vi "resizable_alert_Main.vi"() -> ()   [LabVIEW 2016]
doc: "This template is for the Queued Message Handler design pattern.\n\nThe Event Handling Loop generates messages based on user interface actions.\n\nThe Message Handling Loop processes messages generated by the Event Handling Loop, or by other messages. The messages are string values, so new messages can be added easily to the Message Cases case structure in the Message Handling Loop. Each message cluster can also provide an optional value for Message Data, which is a variant that can be converted to whatever message-specific data is required."
uses:
  controls/resizable_alert_UI Data.ctl
  support/Message Queue/resizable_alert_Message Queue.lvlib
  <vilib>/Utility/error.llb/Error Cluster From Error Code.vi
  support/User Event - Stop/resizable_alert_User Event - Stop.lvlib
  support/Message Queue/Enqueue Message (Single).vi
  <vilib>/ErrorRing/Error Ring.xnode
panel:
  in  "header":string="Header Text"
  in  "explanatory text":string="A brief explanation of what happened and what you can do next."
  in  "close":bool
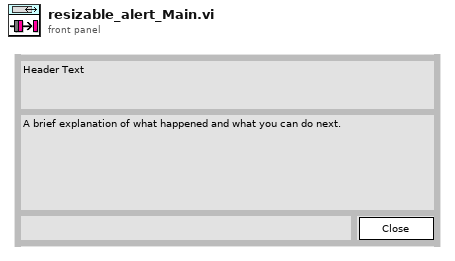
[diagram p1: front panel]
types:
  T1 = typedef "resizable_alert_UI Data.ctl" = cluster{"Exit Button Ref":refnum<vi>}
  T2 = typedef "resizable_alert_Message Queue.lvlib/All Message Queues.ctl" = cluster{"UI":refnum<queue>}
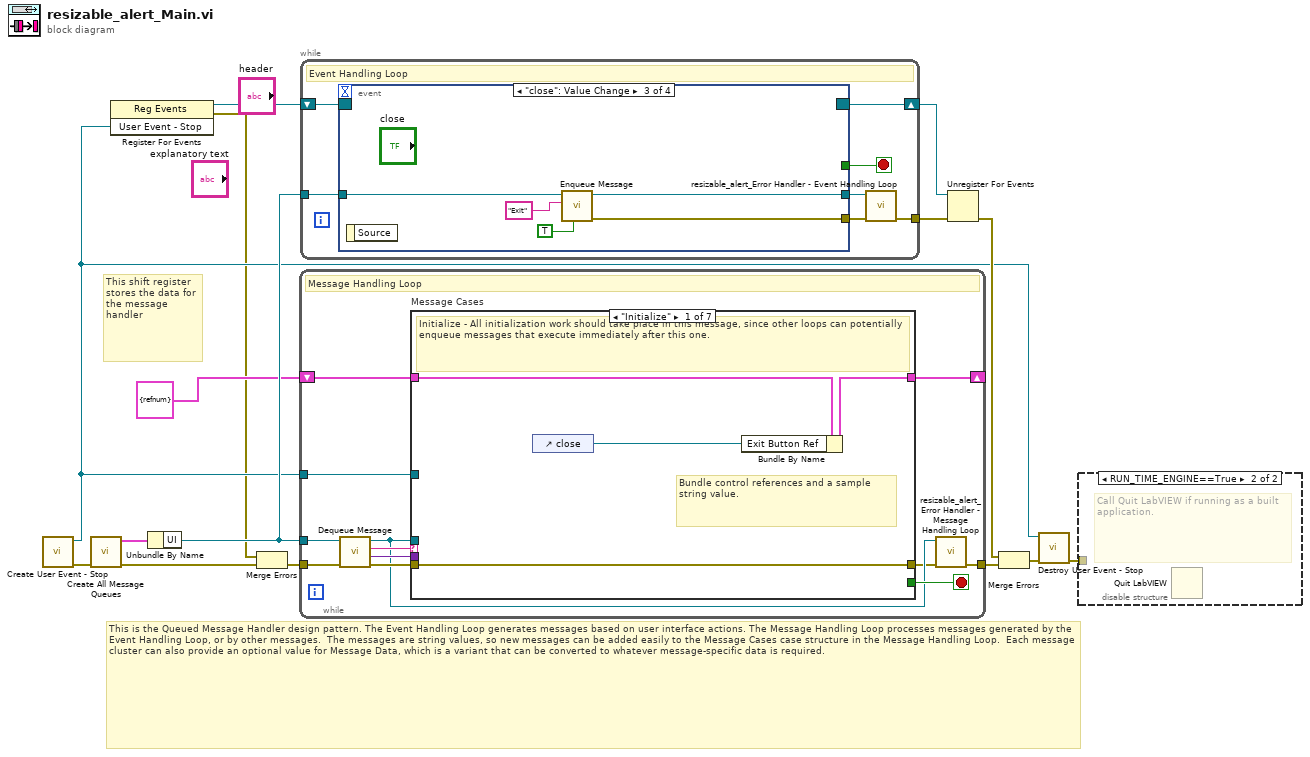
[diagram p0: block diagram]
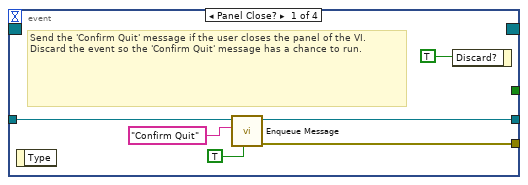
[diagram p3: hidden frame]
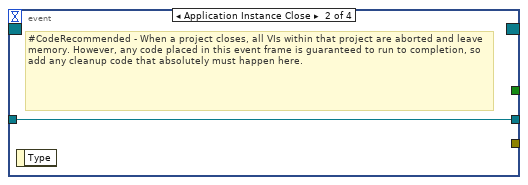
[diagram p4: hidden frame]
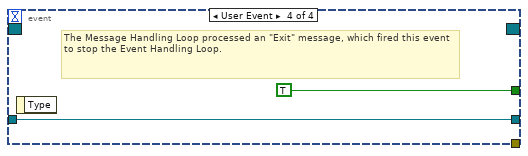
[diagram p5: hidden frame]
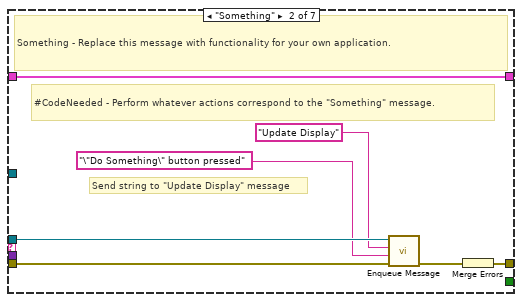
[diagram p6: hidden frame]
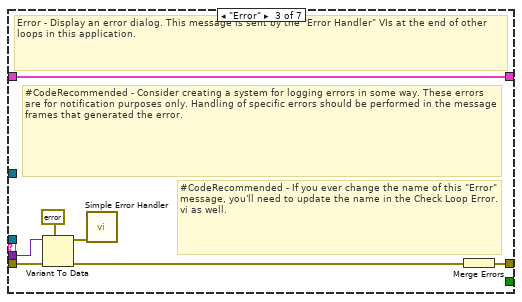
[diagram p7: hidden frame]
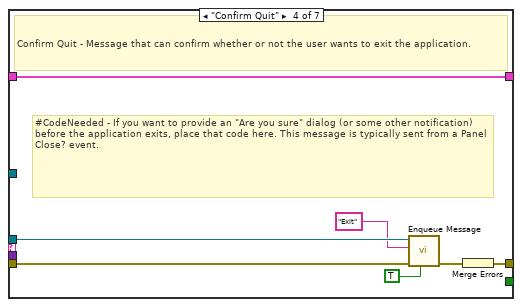
[diagram p8: hidden frame]
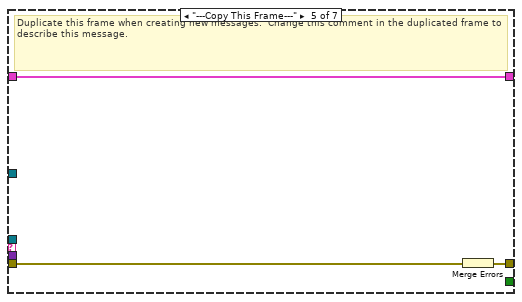
[diagram p9: hidden frame]
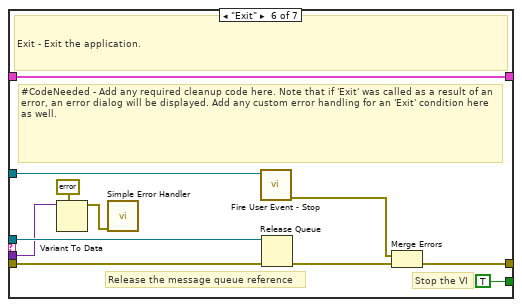
[diagram p10: hidden frame]
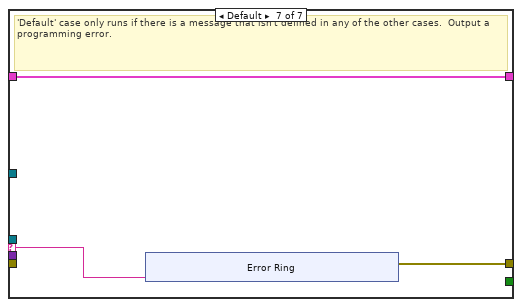
[diagram p11: hidden frame]
diagram:
  # "This is the Queued Message Handler design pattern. The Event Handling Loop generates messages based on user interface actions. The Message Handling Loop processes messages generated by the Event Handling Loop, or by other messages.  The messages are string values, so new messages can be added easily to the Message Cases case structure in the Message Handling Loop.  Each message cluster can also provide an optional value for Message Data, which is a variant that can be converted to whatever message-specific data is required."
  # "This shift register stores the data for the message handler"
  n1 = call "Create User Event - Stop.vi"() -> ("error out"=w11:errorcluster, "User Event - Stop"=w3:refnum<user-event>)  [unwired: 10 in]
  n2 = call "Create All Message Queues.vi"("error in (no error)"=w11) -> ("error out"=w15:errorcluster, "Message Queues out"=w14:T2)  [unwired: 9 in]
  n3 = register-events(w3) -> (reference out=w4:refnum<event-registration>, error out=w1:errorcluster)  [unwired: 2 in]
  n4 = Unbundle By Name(w14) -> ("UI"=w12:refnum<queue>)
  n5 = Merge Errors(w1, w15) -> (w2:errorcluster)
  n6 = while {
    tunnel: w12 -> [w19]
    shift-right: [w26] -> _
    shift-left: T1 {"Exit Button Ref"=refnum} ("Data Cluster") -> [w27]
    tunnel: w3 -> [w24]
    tunnel: w2 -> [w23]
    tunnel: [w17] -> w13
    stop <- w25 stop-if-true
    # "Message Handling Loop"
    n7 = call "Dequeue Message.vi"("error in (no error)"=w23, "Message Queue"=w19) -> ("error out"=w22:errorcluster, "Message Data"=w20:variant, "Message"=w21:string, "dup Message Queue"=w18:refnum<queue>)  [unwired: 6 in]
    n8 = case "Message Cases" shown="\"Initialize\"" w21 {
      selector: w21 -> [_ _ _ _ _ _ w67]
      tunnel: w18 -> [_ w34 _ w48 _ w66 _]
      tunnel: w22 -> [w28 w36 w45 w52 w55 w59 _]
      tunnel: [w28 w37 w39 w50 w53 w62 w68] -> w16
      tunnel: w27 -> [w31 w38 w44 w51 w54 w65 w69]
      tunnel: [w30 w38 w44 w51 w54 w65 w69] -> w26
      tunnel: [_ _ _ _ _ TRUE _] -> w25
      tunnel: w20 -> [_ _ w43 _ _ w56 _]
      tunnel: w24 -> [_ _ _ _ _ w61 _]
      frame "Initialize" {
        # "Bundle control references and a sample string value."
        # "Initialize - All initialization work should take place in this message, since other loops can potentially enqueue messages that execute immediately after this one."
        n9 = control-ref of="close"() -> (w29:refnum<vi>)
        n10 = Bundle By Name(cluster=w31, "Exit Button Ref"=w29) -> (w30:T1)
      }
      frame "Something" {
        # "Send string to \"Update Display\" message"
        # "#CodeNeeded - Perform whatever actions correspond to the \"Something\" message."
        # "Something - Replace this message with functionality for your own application."
        n11 = call-poly "Enqueue Message.vi"("error in (no error)"=w36, "Message Data"="\"Do Something\" button pressed" ("\"Do Something\" button pressed"), "Message"="Update Display", "Message Queue"=w34) -> ("error out"=w35:errorcluster)  [unwired: 6 in, 1 out]
        n12 = Merge Errors(w35) -> (w37:errorcluster)
      }
      frame "Error" {
        # "#CodeRecommended - If you ever change the name of this \"Error\" message, you'll need to update the name in the Check Loop Error.vi as well."
        # "#CodeRecommended - Consider creating a system for logging errors in some way. These errors are for notification purposes only. Handling of specific errors should be performed in the message frames that generated the error."
        # "Error - Display an error dialog. This message is sent by the \"Error Handler\" VIs at the end of other loops in this application."
        n13 = Variant To Data(error in=w45, type=errorcluster {"status"=FALSE, "code"=0, "source"=""} ("error constant"), Variant=w43) -> (data=w41:errorcluster, error out=w40:errorcluster)
        n14 = call <vilib>:"Simple Error Handler.vi"("error in (no error)"=w41) -> ()  [unwired: 4 in, 5 out]
        n15 = Merge Errors(w40) -> (w39:errorcluster)
      }
      frame "Confirm Quit" {
        # "#CodeNeeded - If you want to provide an \"Are you sure\" dialog (or some other notification) before the application exits, place that code here. This message is typically sent from a Panel Close? event."
        # "Confirm Quit - Message that can confirm whether or not the user wants to exit the application."
        n16 = call-poly "Enqueue Message.vi"("Priority Message? (F)"=TRUE, "error in (no error)"=w52, "Message"="Exit", "Message Queue"=w48) -> ("error out"=w49:errorcluster)  [unwired: 6 in, 1 out]
        n17 = Merge Errors(w49) -> (w50:errorcluster)
      }
      frame "---Copy This Frame---" {
        # "Duplicate this frame when creating new messages.  Change this comment in the duplicated frame to describe this message."
        n18 = Merge Errors(w55) -> (w53:errorcluster)
      }
      frame "Exit" {
        # "Stop the VI"
        # "Release the message queue reference"
        # "#CodeNeeded - Add any required cleanup code here. Note that if 'Exit' was called as a result of an error, an error dialog will be displayed. Add any custom error handling for an 'Exit' condition here as well."
        # "Exit - Exit the application."
        n19 = Variant To Data(type=errorcluster {"status"=FALSE, "code"=0, "source"=""} ("error constant"), Variant=w56) -> (data=w57:errorcluster)  [unwired: 1 in, 1 out]
        n20 = call <vilib>:"Simple Error Handler.vi"("error in (no error)"=w57) -> ()  [unwired: 4 in, 5 out]
        n21 = call "Fire User Event - Stop.vi"("User Event - Stop"=w61) -> ("error out"=w60:errorcluster)  [unwired: 10 in]
        n22 = Release Queue(queue=w66, error in (no error)=w59) -> (error out=w63:errorcluster)  [unwired: 1 in, 2 out]
        n23 = Merge Errors(w60, w63) -> (w62:errorcluster)
      }
      frame Default {
        # "'Default' case only runs if there is a message that isn't defined in any of the other cases.  Output a programming error."
        n24 = xnode "Error Ring"("parameter 0"=w67) -> ("error out"=w68:errorcluster)
      }
    }
    n25 = call "resizable_alert_Error Handler - Message Handling Loop.vi"("error in (no error)"=w16, "Message Queue"=w18) -> ("dup error in"=w17:errorcluster)  [unwired: 8 in, 1 out]
  }
  n26 = while {
    tunnel: w12 -> [w83]
    shift-right: [w81] -> w8
    shift-left: w4 -> [w82]
    tunnel: [w77] -> w5
    stop <- w79 stop-if-true
    # "Event Handling Loop"
    n27 = event shown="[2] \"close\": Value Change" {
      selector: w82 -> [_ _ _ _]
      dyn-events: [_ _ _ _] -> w81
      timeout: _ -> [_ _ _ _]
      tunnel: [_ _ _ TRUE ("Discard?")] -> w79
      tunnel: w83 -> [w88 w90 w95 w97]
      tunnel: [w87 _ w94 _] -> w80
      tunnel: [w86 w90 w93 w97] -> w78
      event Panel Close? {
        # "Send the 'Confirm Quit' message if the user closes the panel of the VI. Discard the event so the 'Confirm Quit' message has a chance to run."
        n28 = event-data() -> ()  [unwired: 1 in, 1 out]
        n29 = call-poly "Enqueue Message.vi"("Priority Message? (F)"=TRUE, "Message"="Confirm Quit", "Message Queue"=w88) -> ("error out"=w87:errorcluster, "dup Message Queue"=w86:refnum<queue>)  [unwired: 7 in]
        n30 = event-data("Discard?"=TRUE) -> ()  [unwired: 1 in, 1 out]
      }
      event Application Instance Close {
        # "#CodeRecommended - When a project closes, all VIs within that project are aborted and leave memory. However, any code placed in this event frame is guaranteed to run to completion, so add any cleanup code that absolutely must happen here."
        n31 = event-data() -> ()  [unwired: 1 in, 1 out]
      }
      event "close": Value Change {
        n32 = event-data() -> ()  [unwired: 1 in, 1 out]
        n33 = call-poly "Enqueue Message.vi"("Priority Message? (F)"=TRUE, "Message"="Exit", "Message Queue"=w95) -> ("error out"=w94:errorcluster, "dup Message Queue"=w93:refnum<queue>)  [unwired: 7 in]
      }
      event User Event {
        # "The Message Handling Loop processed an \"Exit\" message, which fired this event to stop the Event Handling Loop."
        n34 = event-data() -> ()  [unwired: 1 in, 1 out]
      }
    }
    n35 = call "resizable_alert_Error Handler - Event Handling Loop.vi"("error in (no error)"=w80, "Message Queue"=w78) -> ("dup error in"=w77:errorcluster)  [unwired: 8 in, 1 out]
  }
  n36 = Unregister For Events(event registration refnum=w8, error in=w5) -> (error out=w9:errorcluster)
  n37 = Merge Errors(w9, w13) -> (w10:errorcluster)
  n38 = call "Destroy User Event - Stop.vi"("error in (no error)"=w10, "User Event - Stop"=w3) -> ("error out"=w6:errorcluster)  [unwired: 9 in]
  n39 = disable-structure shown="RUN_TIME_ENGINE==True" {
    disable-tunnel: w6 -> [_ _]
    frame condition #0 (active) {
    }
    frame condition #1 {
      # "Call Quit LabVIEW if running as a built application."
      n40 = Quit LabVIEW() -> ()  [unwired: 1 in]
    }
  }
